vi "step ac charge test.vi"(8 "error in":errorcluster) -> (0 "error out":errorcluster)   [LabVIEW 2020]
uses:
  <vilib>/AKKA/PROVEtech-RBS/PROVEtechRBS.lvlib
  <vilib>/AKKA/PROVEtech-RBS/SubVIs/Write (Signals Single-point).vi
  <vilib>/AKKA/PROVEtech-RBS/SubVIs/Read (Signals Single-point).vi
panel:
  out "receive unit":string[](array[string])
  out "pass":bool
  out "Array out":string[](array[string])
  out "receive signals":string[](array[string])
  out "sgl array":dbl[](array[numeric])
  out "send unit":string[](array[string])
  out "send values":string[](array[string])
  out "send signals":string[](array[string])
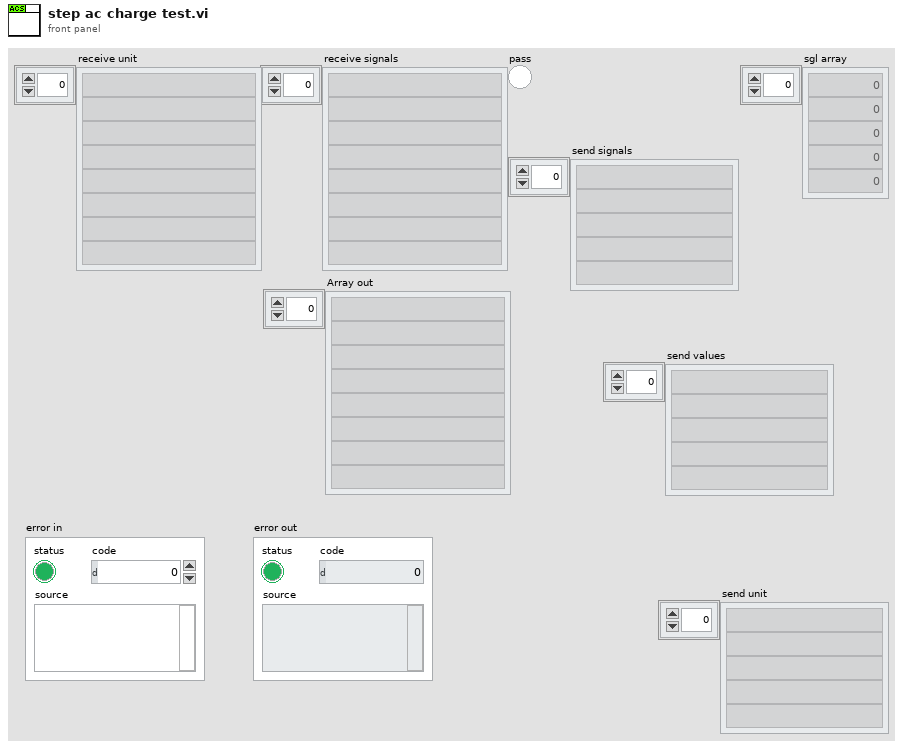
[diagram p1: front panel]
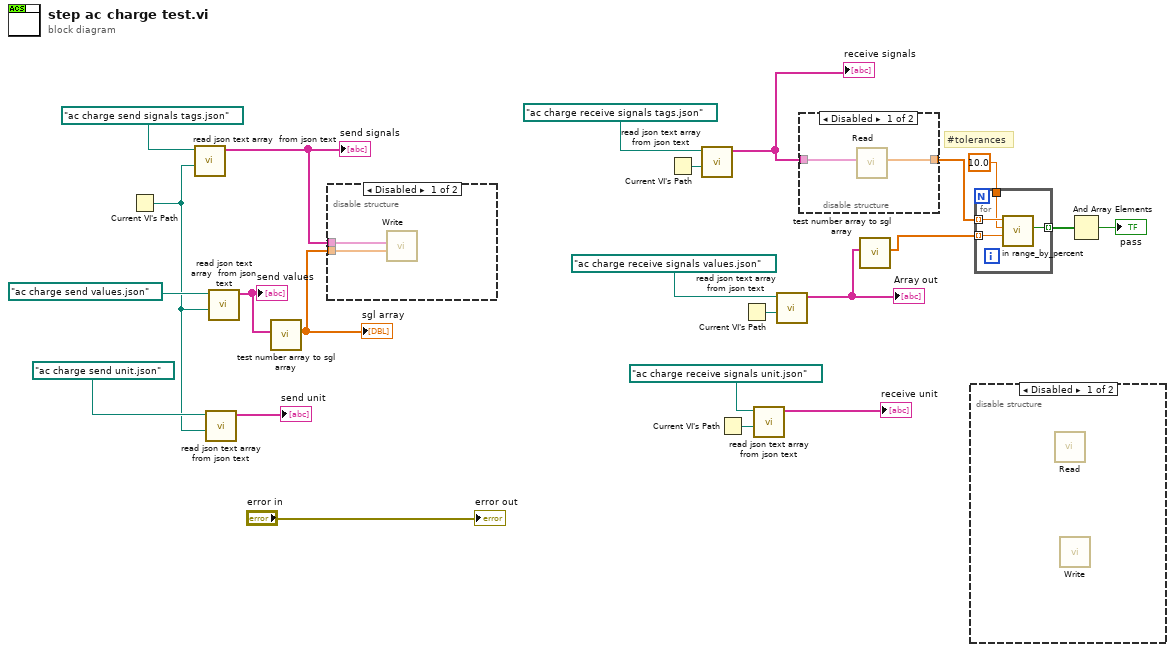
[diagram p0: block diagram]
diagram:
  # "#tolerances"
  n1 = Current VI's Path() -> (path=w2:path)
  n2 = call "read json text array  from json text.vi"("this vis path"=w2, "file name"=path "ac charge send signals tags.json" ("name or relative path")) -> ("Array out"=w18:string[])  [unwired: 8 in, 1 out]
  "send signals" <- w18
  n3 = call "read json text array  from json text.vi"("this vis path"=w2, "file name"=path "ac charge send unit.json" ("name or relative path")) -> ("Array out"=→"send unit":string[])  [unwired: 8 in, 1 out]
  n4 = call "read json text array  from json text.vi"("this vis path"=w2, "file name"=path "ac charge send values.json" ("name or relative path")) -> ("Array out"=w19:string[])  [unwired: 8 in, 1 out]
  "send values" <- w19
  n5 = call "test number array to sgl array.vi"("send values"=w19) -> ("sgl array"=w17:dbl[])  [unwired: 10 in]
  "sgl array" <- w17
  n6 = disable-structure shown="Disabled" {
    disable-tunnel: w18 -> [w25 _]
    disable-tunnel: w17 -> [w24 _]
    frame Disabled {
      n7 = call-poly <vilib>:"Write.vi"("values"=w24, "signals"=w25) -> ()  [unwired: 8 in, 2 out]
    }
    frame Enabled {
    }
  }
  n8 = Current VI's Path() -> (path=w15:path)
  n9 = call "read json text array  from json text.vi"("this vis path"=w15, "file name"=path "ac charge receive signals tags.json" ("name or relative path")) -> ("Array out"=w11:string[])  [unwired: 8 in, 1 out]
  "receive signals" <- w11
  n10 = Current VI's Path() -> (path=w5:path)
  n11 = Current VI's Path() -> (path=w13:path)
  n12 = call "read json text array  from json text.vi"("this vis path"=w5, "file name"=path "ac charge receive signals unit.json" ("name or relative path")) -> ("Array out"=→"receive unit":string[])  [unwired: 8 in, 1 out]
  n13 = call "read json text array  from json text.vi"("this vis path"=w13, "file name"=path "ac charge receive signals values.json" ("name or relative path")) -> ("Array out"=w12:string[])  [unwired: 8 in, 1 out]
  "Array out" <- w12
  n14 = disable-structure shown="Disabled" {
    disable-tunnel: w11 -> [w27 _]
    disable-tunnel: [w26 _] -> w10
    frame Disabled {
      n15 = call-poly <vilib>:"Read.vi"("signals"=w27) -> ("values"=w26:dbl[])  [unwired: 8 in, 2 out]
    }
    frame Enabled {
    }
  }
  n16 = call "test number array to sgl array.vi"("send values"=w12) -> ("sgl array"=w9:dbl[])  [unwired: 10 in]
  n17 = disable-structure shown="Disabled" {
    frame Disabled {
      n18 = call-poly <vilib>:"Read.vi"() -> ()  [unwired: 9 in, 3 out]
      n19 = call-poly <vilib>:"Write.vi"() -> ()  [unwired: 10 in, 2 out]
    }
    frame Enabled {
    }
  }
  n20 = for {
    tunnel: w10 -> [w31] mode=indexing
    tunnel: w9 -> [w30] mode=indexing
    tunnel: 10.0 ("tol %") -> [w29]
    tunnel: [w28] -> w7 mode=indexing
    n21 = call "in range_by_percent.vi"("setpoint"=w30, "tol %"=w29, "x"=w31) -> ("In Range?"=w28:bool)  [unwired: 5 in, 3 out]
  }
  n22 = And Array Elements(Boolean array=w7) -> (logical AND=→"pass":bool)
  "error out" <- "error in"
